vi "SaveControlValues.vi"(7 "Mode":enum16{"Save", "Load"}(ring), 8 "エラー入力":errorcluster, 9 "exception list":string[](array[string]), 10 "file path":path, 11 "Target VI":refnum<vi>) -> (0 "error out":errorcluster, 1 "Value":cluster{"Name":string, "Variant Data":variant}[](array[cluster]), 2 "path":path, 3 "Target VI Out":refnum<vi>)   [LabVIEW 2024]
uses:
  <vilib>/Utility/Data Type/Type Definitions/Data Type.ctl
  <vilib>/Utility/file.llb/Write Delimited Spreadsheet (string).vi
  <vilib>/Utility/Data Type/NI_Data Type.lvlib
panel:
  out "Array":errorcluster[](array[cluster])
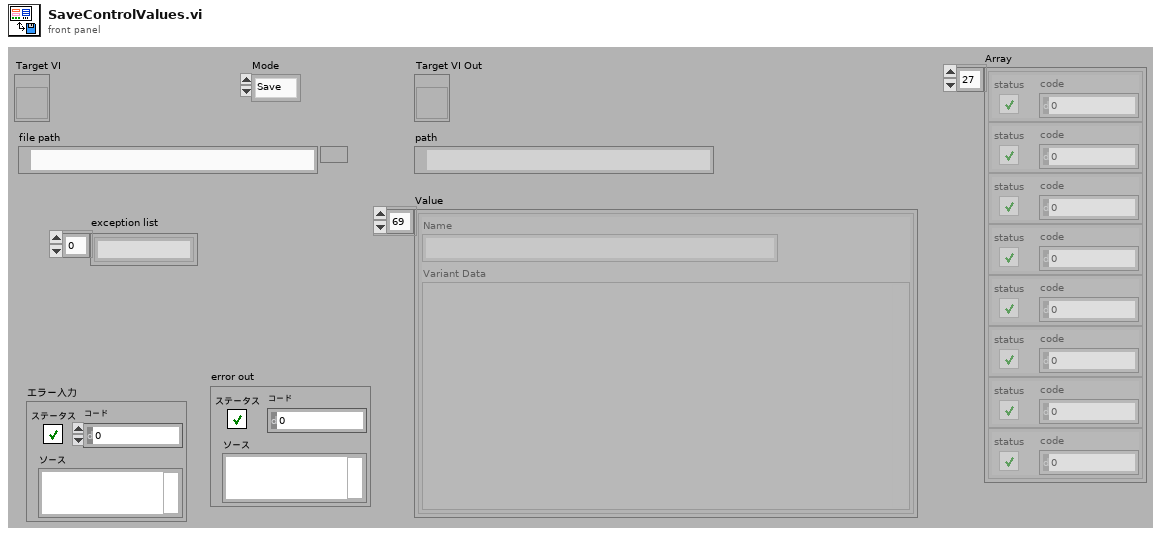
[diagram p1: front panel]
types:
  T1 = enum16{"open", "replace", "create", "open or create", "replace or create", "replace or create with confirmation"}
  T2 = typedef "NI_Data Type.lvlib/Data Type.ctl" = enum8{"Invalid Type", "Void", "I8", "I16", "I32", "I64", "U8", "U16", "U32", "U64", "Single Float", "Double Float", "Extended Float", "Single Complex", "Double Complex", "Extended Complex", "Enum U8", "Enum U16", "Enum U32", "Enum U64", "Single Float With Unit", "Double Float With Unit", "Extended Float With Unit", "Single Complex with Unit", "Double Complex with Unit", "Extended Complex with Unit", "Boolean", "String", "Path", "Picture", "Tag", "Array", "Cluster", "Variant", "LV Variant", "Waveform", "Timestamp", "Digital Waveform", "Digital Data", "ExpressData", "Refnum", "External Data", "VI", "Poly VI", "LabVIEW Class Instance", "Fixed Point", "Set Collection", "Map Collection"}
  T3 = cluster{"Control Value:Get All":cluster{"Name":string, "Variant Data":variant}[]}[]
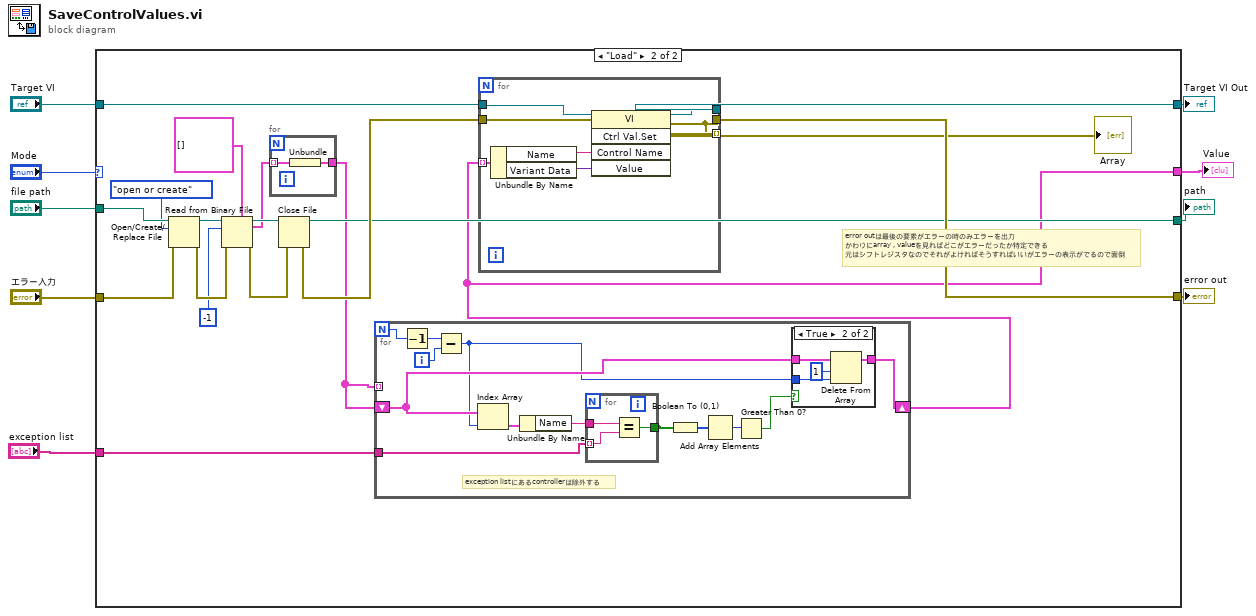
[diagram p0: block diagram]
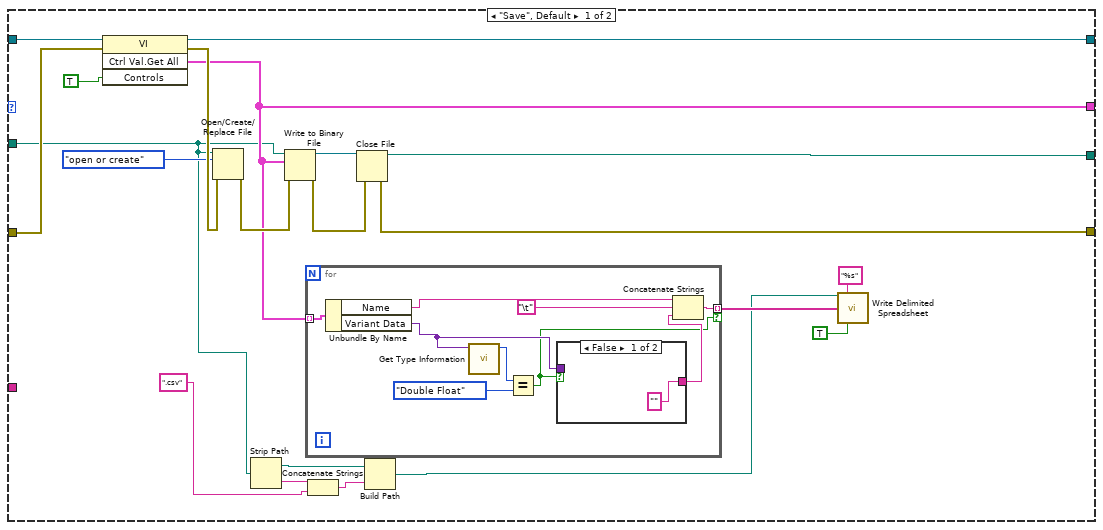
[diagram p2: hidden frame]
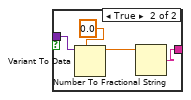
[diagram p3: hidden frame]
diagram:
  n1 = case shown="\"Load\"" "Mode" {
    tunnel: "file path" -> [w16 w63]
    tunnel: "Target VI" -> [w24 w55]
    tunnel: "エラー入力" -> [w23 w56]
    tunnel: [w22 w52] -> w7
    tunnel: [w21 w50] -> w8
    tunnel: [w19 w45] -> w9
    tunnel: [w20 w49] -> w2
    tunnel: "exception list" -> [_ w46]
    frame "Save", Default {
      n2 = invoke class="VI" method="Ctrl Val.Get All"(reference=w24, error in=w23, "Controls"=TRUE) -> (reference out=w20:refnum<vi>, error out=w30:errorcluster, "Get All Control Values Variant"=w19:cluster{"Name":string, "Variant Data":variant}[])  [unwired: 1 in, 1 out]
      n3 = Open/Create/Replace File(file path (use dialog)=w16, error in=w30, operation (0:open)=T1."open or create") -> (error out=w26:errorcluster)  [unwired: 5 out]
      n4 = Strip Path(path=w16) -> (stripped path=w15:path, name=w14:string)
      n5 = Write to Binary File(file (use dialog)=w16, data=w19, error in=w26) -> (refnum out=w27:refnum<file>, error out=w28:errorcluster)  [unwired: 4 out]
      n6 = for {
        tunnel: w19 -> [w39] mode=indexing
        tunnel: [w36] -> w18 mode=indexing if=w31
        n7 = Unbundle By Name(w39) -> ("Name"=w38:string, "Variant Data"=w33:variant)
        n8 = call <vilib>:"Get Type Information.vi"("variant"=w33) -> ("type"=w35:T2)  [unwired: 6 in, 4 out]
        n9 = Equal?(x=w35, y=Data_Type."Double Float" ("type 2")) -> (x = y?=w31:bool)
        n10 = case shown="False" w31 {
          tunnel: w33 -> [_ w44]
          tunnel: ["" w41] -> w32
          frame False {
          }
          frame True {
            n11 = Variant To Data(type=0.0, Variant=w44) -> (data=w42:dbl)  [unwired: 1 in, 1 out]
            n12 = Number To Fractional String(number=w42) -> (F-format string=w41:string)  [unwired: 3 in]
          }
        }
        n13 = Concatenate Strings(w38, "\t", w32) -> (w36:string)
      }
      n14 = Concatenate Strings(w14, ".csv") -> (w12:string)
      n15 = Close File(refnum=w27, error in=w28) -> (path=w21:path, error out=w22:errorcluster)
      n16 = Build Path(base path=w15, name or relative path=w12) -> (appended path=w11:path)
      n17 = call-poly <vilib>:"Write Delimited Spreadsheet.vi"("file path (dialog if empty)"=w11, "format (%s)"="%s", "1D data"=w18, "transpose? (no:F)"=TRUE) -> ()  [unwired: 10 in, 2 out]
    }
    frame "Load" {
      # "error outは最後の要素がエラーの時のみエラーを出力\nかわりにarray , valueを見ればどこがエラーだったか特定できる\n元はシフトレジスタなのでそれがよければそうすればいいがエラーの表示がでるので面倒"
      n18 = Open/Create/Replace File(file path (use dialog)=w63, error in=w56, operation (0:open)=T1."open or create") -> (refnum out=w61:refnum<file>, error out=w60:errorcluster)  [unwired: 4 out]
      n19 = Read from Binary File(5:cluster{"Name":string, "Variant Data":variant}[] [] ("Control Value:Get All"), 8:w60, 10:-1 ("count (1)"), 11:w61) -> (0:w57:errorcluster, 2:w51:T3, 3:w58:refnum<file>)  [unwired: 3 out]
      n20 = for {
        tunnel: w51 -> [w93] mode=indexing
        tunnel: [w92] -> w47
        n21 = Unbundle(w93) -> ("Control Value:Get All"=w92:cluster{"Name":string, "Variant Data":variant}[])
      }
      n22 = Close File(refnum=w58, error in=w57) -> (path=w50:path, error out=w53:errorcluster)
      n23 = for {
        N -> [w76]
        shift-right: [w68] -> w45
        shift-left: w47 -> [w70]
        tunnel: w47 -> [_] mode=indexing
        tunnel: w46 -> [w72]
        i -> [w74]
        # "exception listにあるcontrollerは除外する"
        n24 = Decrement(x=w76) -> (x-1=w75:i32)
        n25 = Subtract(x=w75, y=w74) -> (x-y=w69:i32)
        n26 = Index Array(array=w70, index=w69) -> (element=w73:cluster{"Name":string, "Variant Data":variant})
        n27 = Unbundle By Name(w73) -> ("Name"=w71:string)
        n28 = for {
          tunnel: w72 -> [w83] mode=indexing
          tunnel: w71 -> [w84]
          tunnel: [w82] -> w67 mode=indexing
          tunnel: [w82] -> _
          n29 = Equal?(x=w84, y=w83) -> (x = y?=w82:bool)
        }
        n30 = Boolean To (0,1)(Boolean=w67) -> (0, 1=w66:i16[])
        n31 = Add Array Elements(numeric array=w66) -> (sum=w65:i16)
        n32 = Greater Than 0?(x=w65) -> (x > 0?=w64:bool)
        n33 = case shown="True" w64 {
          tunnel: w70 -> [w77 w81]
          tunnel: w69 -> [_ w80]
          tunnel: [w77 w78] -> w68
          frame False {
          }
          frame True {
            n34 = Delete From Array(array=w81, length=1, index=w80) -> (array with subset deleted=w78:cluster{"Name":string, "Variant Data":variant}[])  [unwired: 1 out]
          }
        }
      }
      n35 = for {
        tunnel: w55 -> [w89]
        tunnel: w45 -> [w88] mode=indexing
        tunnel: [w86] -> w49
        tunnel: w53 -> [w87]
        tunnel: [w85] -> w52
        tunnel: [w85] -> w48 mode=indexing
        n36 = Unbundle By Name(w88) -> ("Name"=w91:string, "Variant Data"=w90:variant)
        n37 = invoke class="VI" method="Ctrl Val.Set"(reference=w89, error in=w87, "Control Name"=w91, "Value"=w90) -> (reference out=w86:refnum<vi>, error out=w85:errorcluster)  [unwired: 1 in, 3 out]
      }
      "Array" <- w48
    }
  }
  "Value" <- w9
  "path" <- w8
  "error out" <- w7
  "Target VI Out" <- w2
